vi "ROI modi and release memory.vi"(7 "reference":refnum<vi>, 11 "beads track":T2[](array[typedef]) {"centroid"."Y Centroid" format="%.2f"; "centroid"."X Centroid" format="%.2f"; "ROI Des out"."Contours"."Type" items=["No Selection", "Point", "Line", "Rectangle", "Oval", "Polygon", "Freehand Region", "Annulus", "Unused2", "Unused3", "Broken Line", "Freehand Line", "Rotated Rectangle"]}) -> ()   [LabVIEW 2017]
uses:
  control/Bead track.ctl
panel:
  out "camera window":T1(plugin-control)
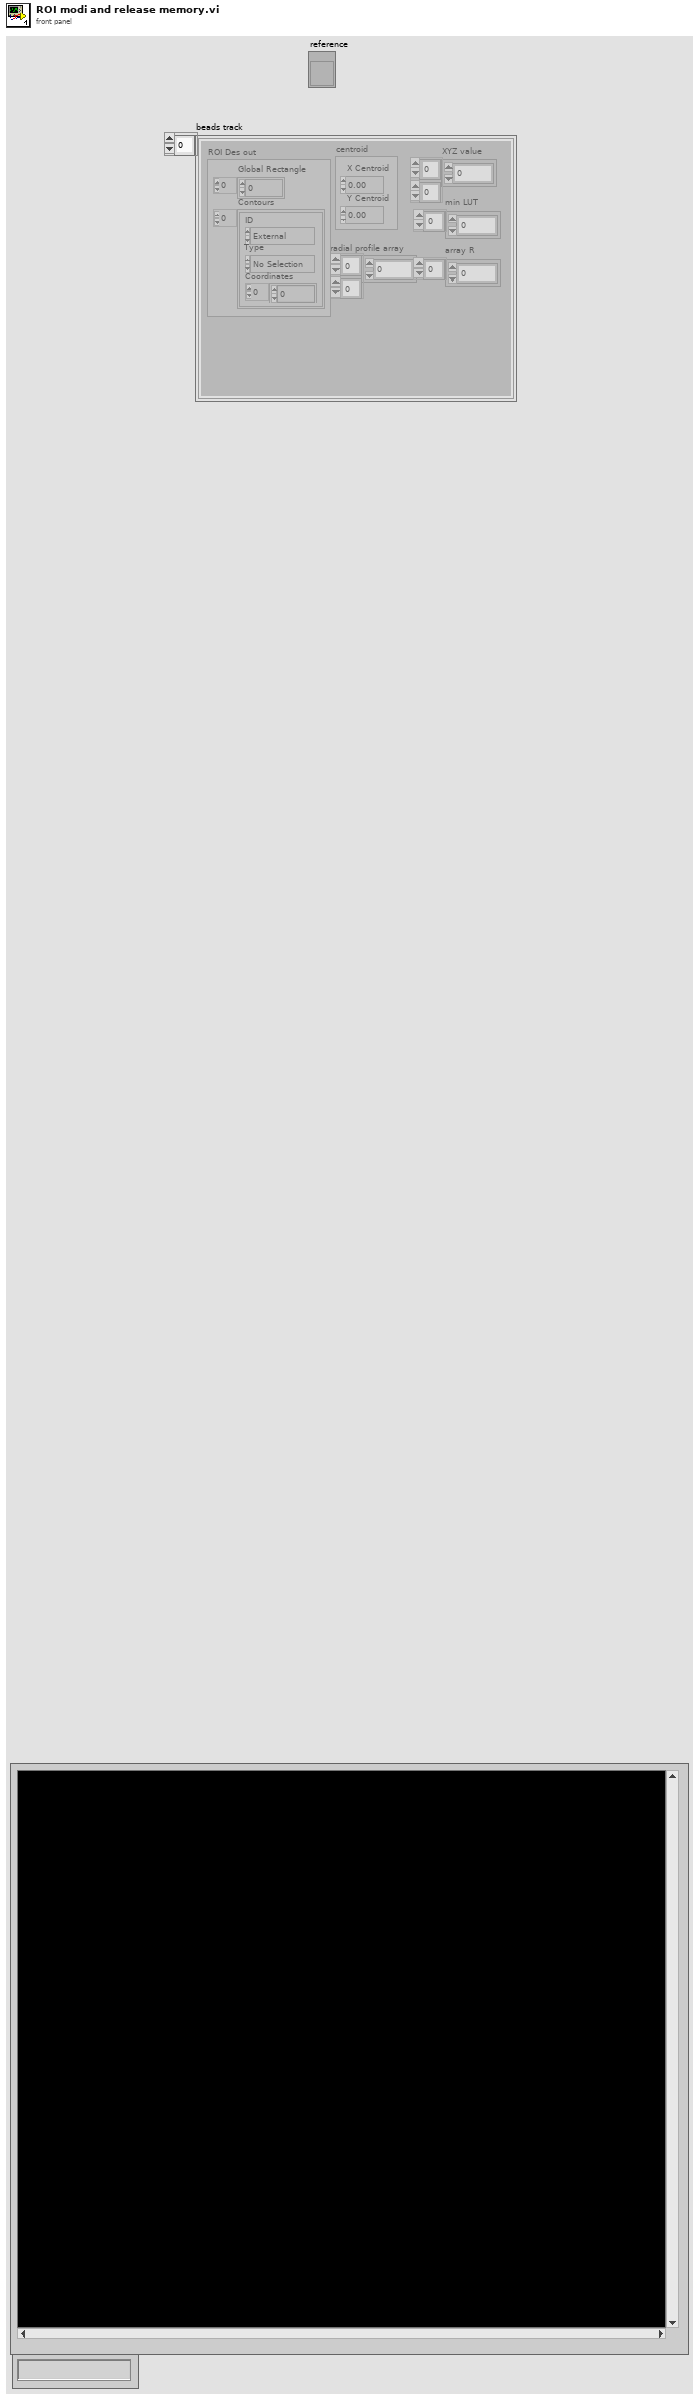
[diagram p1: front panel]
types:
  T1 = typedef "IMAQ Image.ctl" = refnum<image>
  T2 = typedef "Bead track.ctl" = cluster{"XYZ value":dbl[][], "radial profile array":dbl[][], "min LUT":dbl[], "ROI Des out":T3, "array R":dbl[], "centroid":cluster{"X Centroid":sgl, "Y Centroid":sgl}}
  T3 = typedef "ROI Descriptor" = cluster{"Global Rectangle":i32[], "Contours":cluster{"ID":enum32{"External", "Internal"}, "Type":u32, "Coordinates":i32[]}[]}
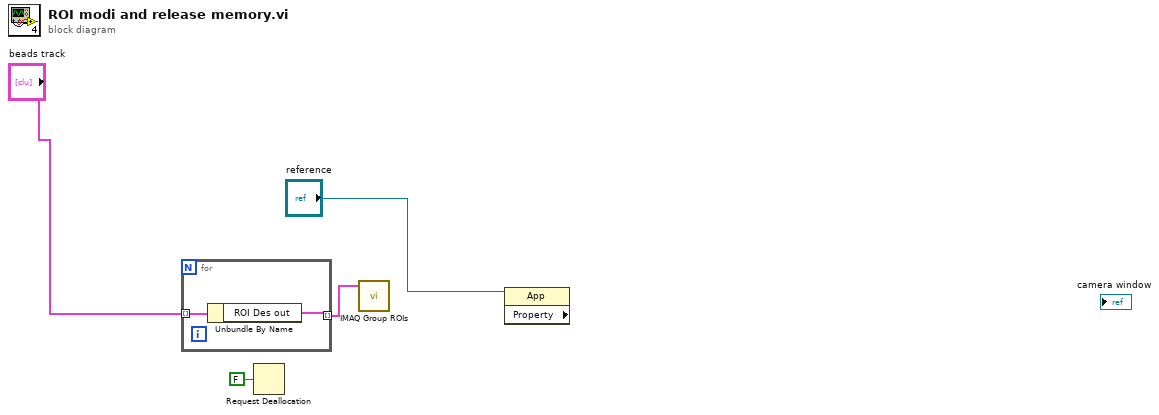
[diagram p0: block diagram]
diagram:
  n1 = for {
    tunnel: [w6] -> w4 mode=indexing
    tunnel: "beads track" -> [w5] mode=indexing
    n2 = Unbundle By Name(w5) -> ("ROI Des out"=w6:T3)
  }
  n3 = Request Deallocation(FALSE ("flag")) -> ()
  n4 = call "IMAQ Group ROIs"("ROI Descriptors"=w4) -> ()  [unwired: 3 in, 2 out]
  n5 = property class="App" props=[](reference="reference") -> ()  [unwired: 1 in, 3 out]
